vi "Read Type.vi"(8 "Error In":errorcluster, 11 "Text In":refnum<class "Text.lvclass">) -> (0 "Error Out":errorcluster, 2 "Type":T1=enum."Unknown", 3 "Text Out":refnum<class "Text.lvclass">)   [LabVIEW 2018, in "Toolkit.lvlib" / "Tokens.lvlib" / "Text.lvclass"]
doc: "Gets the Token type of an object. This is primarily used internally or when building custom compilers. This is more robust than using strings in case structures with the Get LV Class Name function, which is not available in older versions of LabVIEW.\n\n<B>Text In/Out</B> - Represents an identified token from a lexed Mustache template.\n\n<B>Type</B> - Indicates the token's type as an enum."
uses:
  Text.lvclass
  Type Definitions/Types.ctl
  Tokens.lvlib
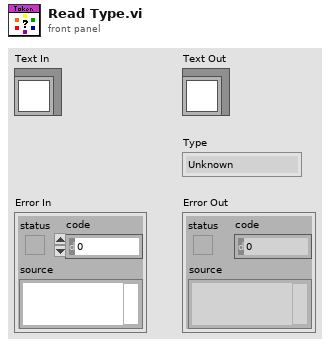
[diagram p1: front panel]
types:
  T1 = typedef "Toolkit.lvlib/Tokens.lvlib/Types.ctl" = enum16{"Begin Section", "Comment", "End Section", "Escaped Variable", "Inverted Section", "Partial", "Set Delimiter", "Text", "Unescaped Variable", "Unknown"}
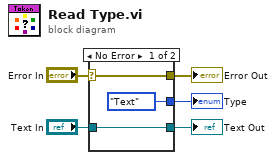
[diagram p0: block diagram]
diagram:
  n1 = case shown="No Error" "Error In" {
    selector: "Error In" -> [w8 w9]
    tunnel: [w8 w9] -> w2
    tunnel: "Text In" -> [w7 w10]
    tunnel: [w7 w10] -> w3
    tunnel: [Types."Text" ("Type") _] -> w1
    frame No Error {
    }
    frame Error {
    }
  }
  "Error Out" <- w2
  "Text Out" <- w3
  "Type" <- w1
